vi "Save Video.vi"() -> ()   [LabVIEW 2018]
doc: "Save Video: This sample video saves a video clip that calls the camera in a local file."
uses:
  vi.lib/VIRobotics/opencv_yiku/ctls/ColorConversionCodes.ctl
  vi.lib/VIRobotics/opencv_yiku/Mat/Mat_8U/Mat_8U.lvclass
  D:/Program Files/company/National Instruments/LabVIEW 2018/vi.lib/addons/VIRobotics/opencv_yiku/Mat/Mat/Mat.lvclass
  vi.lib/VIRobotics/opencv_yiku/Mat/Create_Mat_8U.vi
  vi.lib/VIRobotics/opencv_yiku/Cap/setFPS.vi
  vi.lib/VIRobotics/opencv_yiku/VideoWriter/VideoWriter_release.vi
  vi.lib/VIRobotics/opencv_yiku/Cap/Cap.lvclass
  vi.lib/VIRobotics/opencv_yiku/opencv_yiku.lvlib
  vi.lib/VIRobotics/opencv_yiku/VideoWriter/VideoWriter.lvclass
panel:
  out "time":u32
  in  "stop":bool
  out "picture":picture
  in  "Width":dbl=640.0
  in  "Height":dbl=480.0
  in  "URL":string="rtmp://ns8.indexforce.com/home/mystream"
  in  "Source":enum16{"cameraID", "URL"}(ring)
  in  "cameraID":i32
  # "Overview: Demonstrates how to save the video\nRequirements: Windows.\nInstructions: \n1. Run the VI\n2.Make sure your computer has a camera"
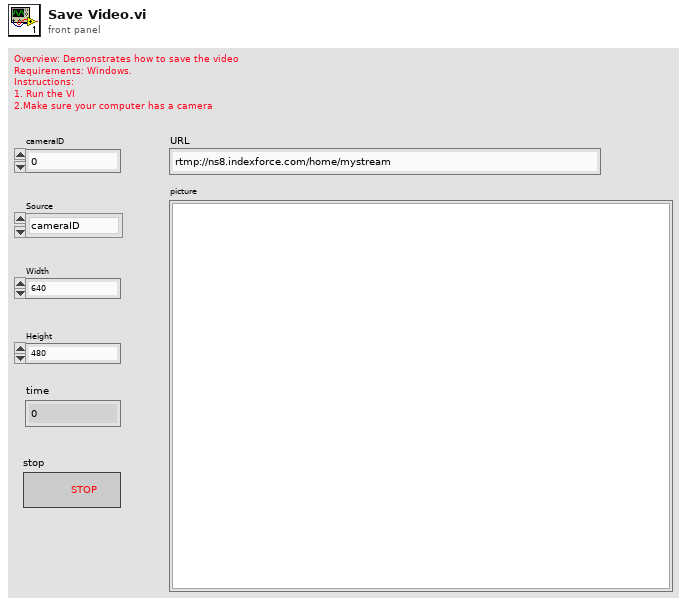
[diagram p1: front panel]
types:
  T1 = typedef "opencv_yiku.lvlib/ColorConversionCodes.ctl" = enum32{"COLOR_BGR2BGRA", "COLOR_BGRA2BGR", "COLOR_BGR2RGBA", "COLOR_RGBA2BGR", "COLOR_BGR2RGB", "COLOR_BGRA2RGBA", "COLOR_BGR2GRAY", "COLOR_RGB2GRAY", "COLOR_GRAY2BGR", "COLOR_GRAY2BGRA", "COLOR_BGRA2GRAY", "COLOR_RGBA2GRAY", "COLOR_BGR2BGR565", "COLOR_RGB2BGR565", "COLOR_BGR5652BGR", "COLOR_BGR5652RGB", "COLOR_BGRA2BGR565", "COLOR_RGBA2BGR565", "COLOR_BGR5652BGRA", "COLOR_BGR5652RGBA", "COLOR_GRAY2BGR565", "COLOR_BGR5652GRAY", "COLOR_BGR2BGR555", "COLOR_RGB2BGR555", "COLOR_BGR5552BGR", "COLOR_BGR5552RGB", "COLOR_BGRA2BGR555", "COLOR_RGBA2BGR555", "COLOR_BGR5552BGRA", "COLOR_BGR5552RGBA", "COLOR_GRAY2BGR555", "COLOR_BGR5552GRAY", "COLOR_BGR2XYZ", "COLOR_RGB2XYZ", "COLOR_XYZ2BGR", "COLOR_XYZ2RGB", "COLOR_BGR2YCrCb", "COLOR_RGB2YCrCb", "COLOR_YCrCb2BGR", "COLOR_YCrCb2RGB", "COLOR_BGR2HSV", "COLOR_RGB2HSV", "42", "43", "COLOR_BGR2Lab", "COLOR_RGB2Lab"}
  T2 = typedef "LVBoundsTypeDef.ctl" = cluster{"Width":u32, "Height":u32}
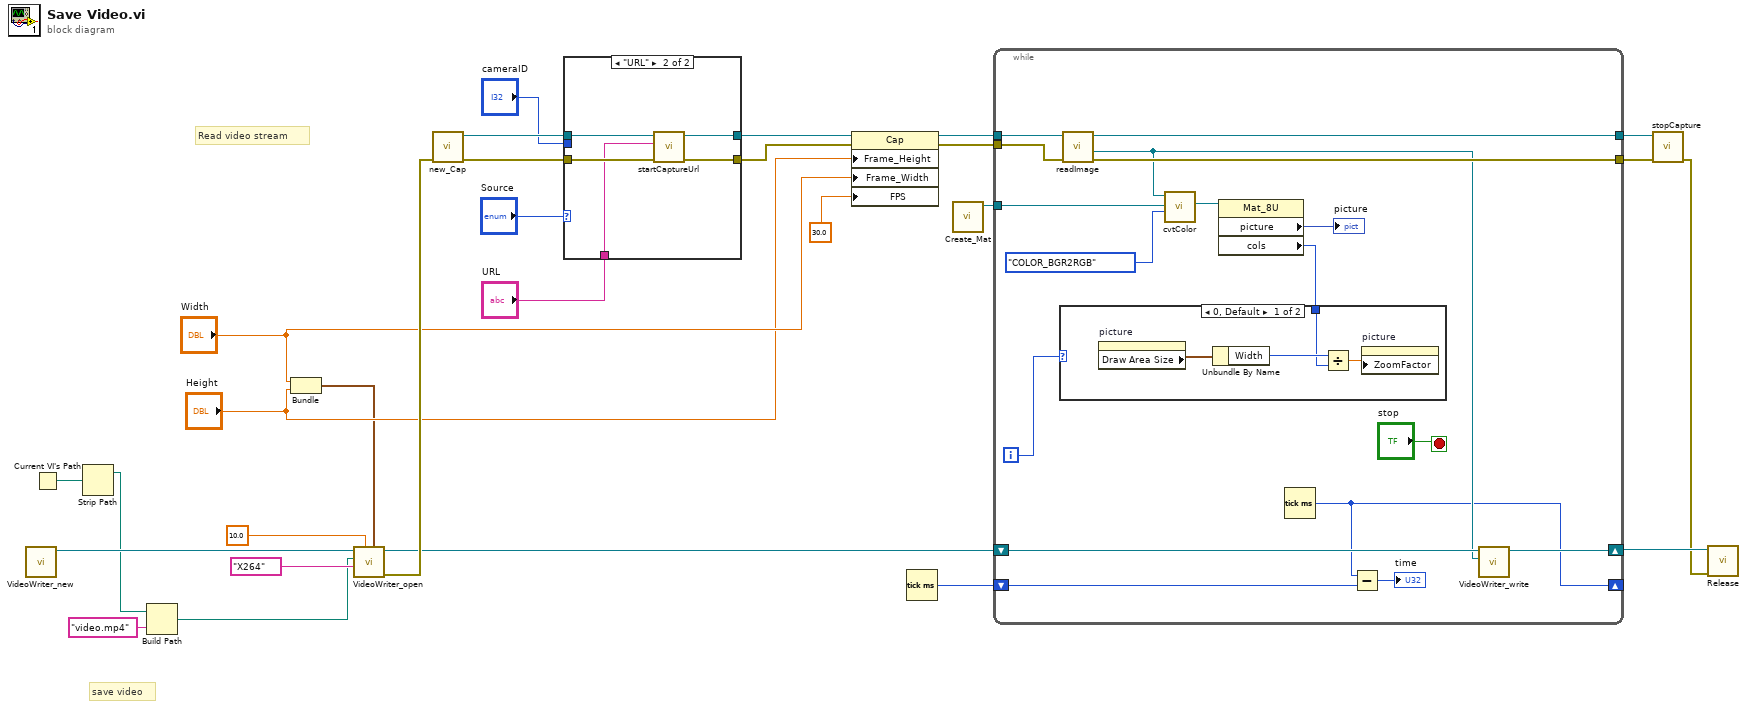
[diagram p0: block diagram]
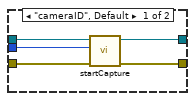
[diagram p3: hidden frame]
diagram:
  # "save video"
  # "Read video stream"
  n1 = call "VideoWriter_new.vi"() -> ("VideoWriter out"=w17:refnum<class "VideoWriter.lvclass">)  [unwired: 10 in, 1 out]
  n2 = Current VI's Path() -> (path=w4:path)
  n3 = Strip Path(path=w4) -> (stripped path=w3:path)  [unwired: 1 out]
  n4 = Build Path(base path=w3, name or relative path="video.mp4") -> (appended path=w13:path)
  n5 = Bundle("Width"="Width", "Height"="Height") -> (w9:cluster{"Width":dbl, "Height":dbl})  [unwired: 1 in]
  n6 = call "VideoWriter_open.vi"("Size"=w9, "fps"=10.0, "format"="X264", "filename"=w13, "VideoWriter in"=w17) -> ("error out"=w12:errorcluster, "VideoWriter out"=w8:refnum<class "VideoWriter.lvclass">)  [unwired: 5 in]
  n7 = call "new_Cap.vi"("error in (no error)"=w12) -> ("error out"=w27:errorcluster, "Cap out"=w28:refnum<class "Cap.lvclass">)  [unwired: 9 in]
  n8 = case shown="\"URL\"" "Source" {
    tunnel: w28 -> [w33 w38]
    tunnel: w27 -> [w32 w36]
    tunnel: "cameraID" -> [w31 _]
    tunnel: [w30 w37] -> w23
    tunnel: [w29 w35] -> w22
    tunnel: "URL" -> [_ w34]
    frame "cameraID", Default {
      n9 = call "startCapture.vi"("error in (no error)"=w32, "cameraID"=w31, "Cap in"=w33) -> ("error out"=w29:errorcluster, "Cap out"=w30:refnum<class "Cap.lvclass">)  [unwired: 7 in]
    }
    frame "URL" {
      n10 = call-dynamic "startCaptureUrl.vi"("error in (no error)"=w36, "url"=w34, "Cap in"=w38) -> ("error out"=w35:errorcluster, "Cap out"=w37:refnum<class "Cap.lvclass">)  [unwired: 7 in]
    }
  }
  n11 = property class="Cap"(reference=w23, error in=w22, "Frame_Height"="Height", "Frame_Width"="Width", "FPS"=30.0) -> (reference out=w21:refnum<class "Cap.lvclass">, error out=w20:errorcluster)
  n12 = Tick Count (ms)() -> (millisecond timer value=w1:u32)
  n13 = call-poly "Create_Mat.vi"() -> ("Mat_8U_out"=w7:refnum<class "Mat_8U.lvclass">)  [unwired: 10 in, 1 out]
  n14 = while {
    tunnel: w21 -> [w55]
    tunnel: w20 -> [w54]
    tunnel: [w52] -> w19
    tunnel: [w51] -> w18
    shift-right: [w42] -> w6
    shift-left: w8 -> [w44]
    tunnel: w7 -> [w45]
    shift-right: [w40] -> _
    shift-left: w1 -> [w41]
    i -> [w47]
    stop <- "stop" stop-if-true
    n15 = call "readImage.vi"("error in (no error)"=w54, "Cap in"=w55) -> ("error out"=w51:errorcluster, "Mat out"=w43:refnum<class "Mat_8U.lvclass">, "Cap out"=w52:refnum<class "Cap.lvclass">)  [unwired: 7 in]
    n16 = call "cvtColor.vi"("dstCn"=ColorConversionCodes."COLOR_BGR2RGB", "dst"=w45, "src"=w43) -> ("dst out"=w50:refnum<class "Mat_8U.lvclass">)  [unwired: 6 in, 2 out]
    n17 = property class="Mat_8U"(reference=w50) -> ("picture"=→"picture":picture, "cols"=w46:i32)  [unwired: 1 in, 2 out]
    n18 = case shown="0, Default" w47 {
      tunnel: w46 -> [w57 _]
      frame 0, Default {
        n19 = property on="picture" class="Pict"() -> ("Draw Area Size"=w59:T2)  [unwired: 2 in, 2 out]
        n20 = Unbundle By Name(w59) -> ("Width"=w58:u32)
        n21 = Divide(x=w58, y=w57) -> (x/y=w56:dbl)
        n22 = property on="picture" class="Pict"("ZoomFactor"=w56) -> ()  [unwired: 2 in, 2 out]
      }
      frame 1 {
      }
    }
    n23 = Tick Count (ms)() -> (millisecond timer value=w40:u32)
    n24 = Subtract(x=w40, y=w41) -> (x-y=→"time":u32)
    n25 = call "VideoWriter_write.vi"("img"=w43, "VideoWriter in"=w44) -> ("VideoWriter out"=w42:refnum<class "VideoWriter.lvclass">)  [unwired: 8 in, 1 out]
  }
  n26 = call "stopCapture.vi"("error in (no error)"=w18, "Cap in"=w19) -> ("error out"=w5:errorcluster)  [unwired: 9 in]
  n27 = call-poly "Release.vi"("error in (no error)"=w5, "VideoWriter in"=w6) -> ()  [unwired: 9 in, 1 out]
